vi "Append.vi"(6 "deadline":T1={"mode"=enum."Relative", "deadline (ms)"=30000}, 8 "error in (no error)":errorcluster, 10 "data":u8[](array[numeric]), 11 "File Download Controller in":refnum<class "File Download Controller.lvclass">) -> (0 "error out":errorcluster, 3 "File Download Controller out":refnum<class "File Download Controller.lvclass">)   [LabVIEW 2020, in "NI_SFTP.lvlib" / "File Download Controller.lvclass"]
uses:
  <vilib>/net/SFTP/API/Support/Download/File/File Download Controller.lvclass
  <vilib>/Utility/Deadline/Deadline.ctl
  <vilib>/Utility/Deadline/Mode.ctl
  <vilib>/net/SFTP/API/Support/Download/File/File Download Controller.lvclass/File Download Controller.ctl
  <vilib>/Utility/Deadline/NI_Deadline.lvlib
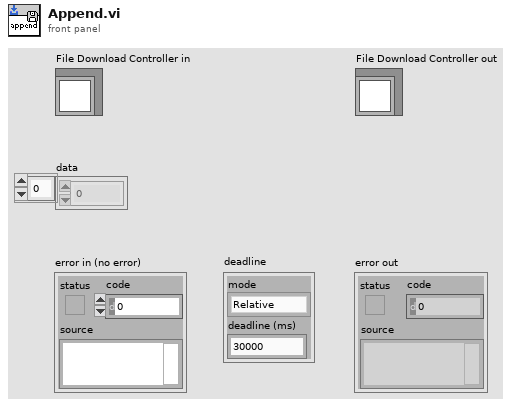
[diagram p1: front panel]
types:
  T1 = typedef "NI_Deadline.lvlib/Deadline.ctl" = cluster{"mode":T2, "deadline (ms)":u32}
  T2 = typedef "NI_Deadline.lvlib/Mode.ctl" = enum16{"Relative", "Use deadline", "Wait forever", "Nonblocking", "N/A"}
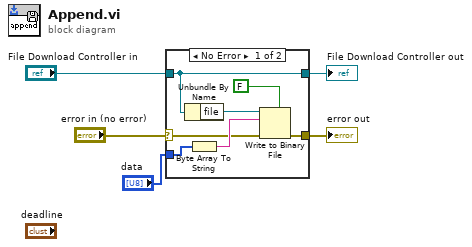
[diagram p0: block diagram]
diagram:
  n1 = case shown="No Error" "error in (no error)" {
    selector: "error in (no error)" -> [w8 w14]
    tunnel: [w7 w14] -> w4
    tunnel: [w12 w13] -> w2
    tunnel: "File Download Controller in" -> [w12 w13]
    tunnel: "data" -> [w10 _]
    frame No Error {
      n2 = Unbundle By Name(w12) -> ("file"=w11:refnum<file>)
      n3 = Byte Array To String(unsigned byte array=w10) -> (string=w9:string)
      n4 = Write to Binary File(file (use dialog)=w11, data=w9, error in=w8, 5:FALSE ("prepend array or string size? (T)")) -> (error out=w7:errorcluster)  [unwired: 2 in, 2 out]
    }
    frame Error {
    }
  }
  "error out" <- w4
  "File Download Controller out" <- w2
